vi "templates style to record parameters.vi"(8 "error in (no error)":errorcluster, 10 "user":string, 11 "template style":string) -> (0 "error out":errorcluster, 2 "Parameters":T2, 3 "Template Record":T1)   [LabVIEW 2011]
uses:
  ITK EXT/utils/keyedarr.llb/Keyed Array.ctl
  server/database/Templates/Template Record.ctl
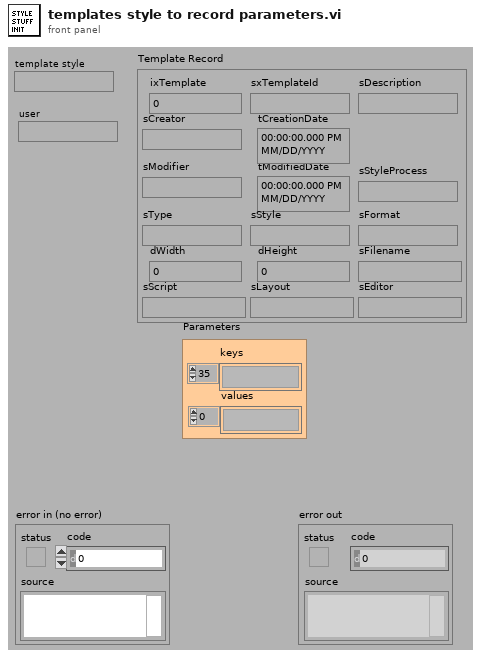
[diagram p1: front panel]
types:
  T1 = typedef "Template Record.ctl" = cluster{"ixTemplate":i32, "sxTemplateId":string, "sDescription":string, "sCreator":string, "tCreationDate":timestamp, "sModifier":string, "tModifiedDate":timestamp, "sType":string, "sStyle":string, "sFormat":string, "dWidth":dbl, "dHeight":dbl, "sFilename":string, "sScript":string, "sLayout":string, "sEditor":string, "sStyleProcess":string}
  T2 = typedef "Keyed Array.ctl" = cluster{"keys":string[], "values":string[]}
  T3 = enum16{"open", "replace", "create", "open or create", "replace or create", "replace or create with confirmation"}
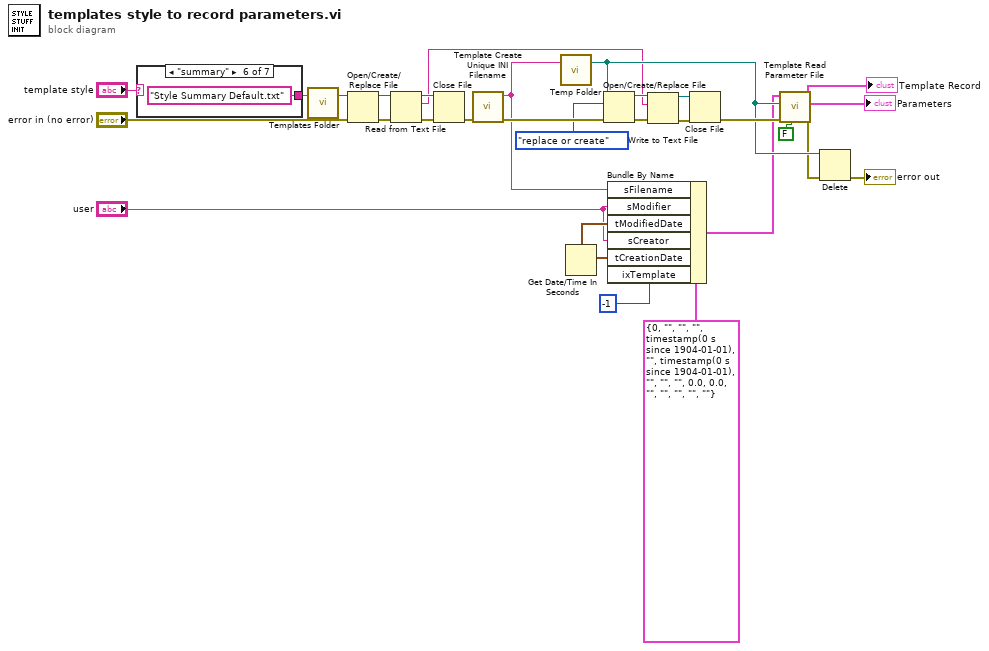
[diagram p0: block diagram]
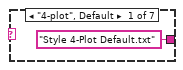
[diagram p2: hidden frame]
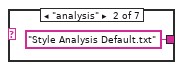
[diagram p3: hidden frame]
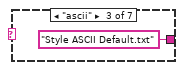
[diagram p4: hidden frame]
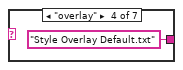
[diagram p5: hidden frame]
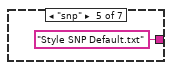
[diagram p6: hidden frame]
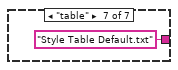
[diagram p7: hidden frame]
diagram:
  n1 = case shown="\"summary\"" "template style" {
    tunnel: ["Style 4-Plot Default.txt" "Style Analysis Default.txt" "Style ASCII Default.txt" "Style Overlay Default.txt" "Style SNP Default.txt" "Style Summary Default.txt" "Style Table Default.txt"] -> w1
    frame "4-plot", Default {
    }
    frame "analysis" {
    }
    frame "ascii" {
    }
    frame "overlay" {
    }
    frame "snp" {
    }
    frame "summary" {
    }
    frame "table" {
    }
  }
  n2 = call "Templates Folder.vi"("Relative Path (\"\")"=w1) -> ("Templates Folder"=w3:path)  [unwired: 2 out]
  n3 = Open/Create/Replace File(file path (use dialog)=w3, error in="error in (no error)") -> (refnum out=w5:refnum<file>, error out=w8:errorcluster)  [unwired: 1 in, 4 out]
  n4 = Read from Text File(file (use dialog)=w5, error in=w8) -> (refnum out=w4:refnum<file>, text=w2:string, error out=w7:errorcluster)  [unwired: 2 in, 1 out]
  n5 = Close File(refnum=w4, error in=w7) -> (error out=w6:errorcluster)  [unwired: 1 out]
  n6 = call "Template Create Unique INI Filename.vi"("error in (no error)"=w6) -> ("error out"=w28:errorcluster, "INI Name"=w11:string)  [unwired: 9 out]
  n7 = call "Temp Folder.vi"("Relative Path (\"\")"=w11) -> ("Temp Folder"=w17:path)  [unwired: 2 in]
  n8 = Get Date/Time In Seconds() -> (seconds since 1Jan1904=w15:timestamp)
  n9 = Open/Create/Replace File(file path (use dialog)=w17, error in=w28, operation (0:open)=T3."replace or create") -> (refnum out=w23:refnum<file>, error out=w24:errorcluster)  [unwired: 4 out]
  n10 = Bundle By Name(cluster=T1 {"ixTemplate"=0, "sxTemplateId"="", "sDescription"="", "sCreator"="", "tCreationDate"=timestamp(0 s since 1904-01-01), "sModifier"="", "tModifiedDate"=timestamp(0 s since 1904-01-01), "sType"="", "sStyle"="", "sFormat"="", "dWidth"=0.0, "dHeight"=0.0, "sFilename"="", "sScript"="", "sLayout"="", "sEditor"="", "sStyleProcess"=""} ("Template Record"), "sFilename"=w11, "sModifier"="user", "tModifiedDate"=w15, "sCreator"="user", "tCreationDate"=w15, "ixTemplate"=-1) -> (w14:T1)
  n11 = Write to Text File(file (use dialog)=w23, text=w2, error in=w24) -> (refnum out=w25:refnum<file>, error out=w26:errorcluster)  [unwired: 2 out]
  n12 = Close File(refnum=w25, error in=w26) -> (error out=w27:errorcluster)  [unwired: 1 out]
  n13 = call "Template Read Parameter File.vi"("Import?"=FALSE, "error in (no error)"=w27, "Alternate Path (\"\")"=w17, "Template Record"=w14) -> ("error out"=w16:errorcluster, "Parameters"=→"Parameters":T2, "updated Template Record"=→"Template Record":T1)  [unwired: 5 out]
  n14 = Delete(path (use dialog)=w17, error in=w16) -> (error out=→"error out":errorcluster)  [unwired: 5 out]
